vi "Delete Edges.vi"(0 "FSM.Graph In":refnum<class "FSM.Graph.lvclass">, 7 "Name":string) -> (4 "FSM.Graph Out":refnum<class "FSM.Graph.lvclass">)   [LabVIEW 2020, in "FSM.Graph.lvclass"]
uses:
  FSM.Graph.lvclass
  FSM.Graph.lvclass/FSM.Graph.ctl
  FSM.Edge/FSM.Edge.lvclass/FSM.Edge.ctl
  FSM.Label/FSM.Label.lvclass/FSM.Label.ctl
  FSM.Edge/Read Label.vi
  FSM.Label/Read Text.vi
  FSM.Edge/FSM.Edge.lvclass
  FSM.Label/FSM.Label.lvclass
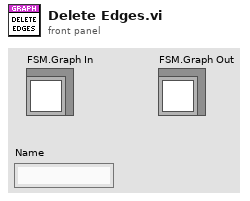
[diagram p1: front panel]
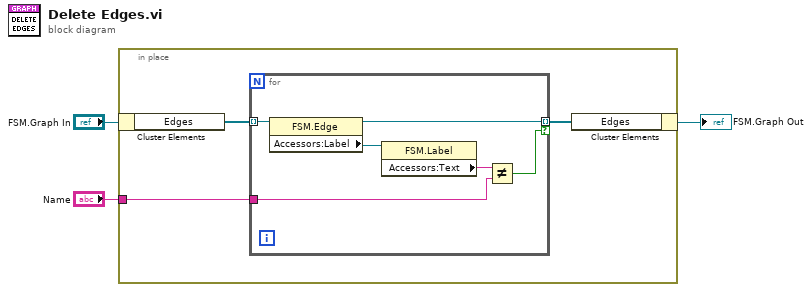
[diagram p0: block diagram]
diagram:
  n1 = in-place {
    in-place-border: "Name" -> [w4]
    n2 = in-place-cluster #1("FSM.Graph In") -> ("Edges"=w6:refnum<class "FSM.Edge.lvclass">[])
    n3 = for {
      tunnel: w6 -> [w12] mode=indexing
      tunnel: [w11] -> w5 mode=indexing if=w8
      tunnel: w4 -> [w7]
      n4 = property class="FSM.Edge"(reference=w12) -> (reference out=w11:refnum<class "FSM.Edge.lvclass">, "Accessors:Label"=w10:refnum<class "FSM.Label.lvclass">)  [unwired: 1 in, 1 out]
      n5 = property class="FSM.Label"(reference=w10) -> ("Accessors:Text"=w9:string)  [unwired: 1 in, 2 out]
      n6 = Not Equal?(x=w9, y=w7) -> (x != y?=w8:bool)
    }
    n7 = in-place-cluster #1("Edges"=w5) -> (→"FSM.Graph Out":refnum<class "FSM.Graph.lvclass">)
  }
